vi "String.Merge data from 2 lists.vi"(8 "New Values":string[](array[string]), 9 "New Names":string[](array[string]), 11 "Names":string[](array[string])) -> (1 "Added Names":bool, 2 "Values Out":string[](array[string]), 3 "Names Out":string[](array[string]))   [LabVIEW 2019]
panel:
  out "appended array":string[](array[string])
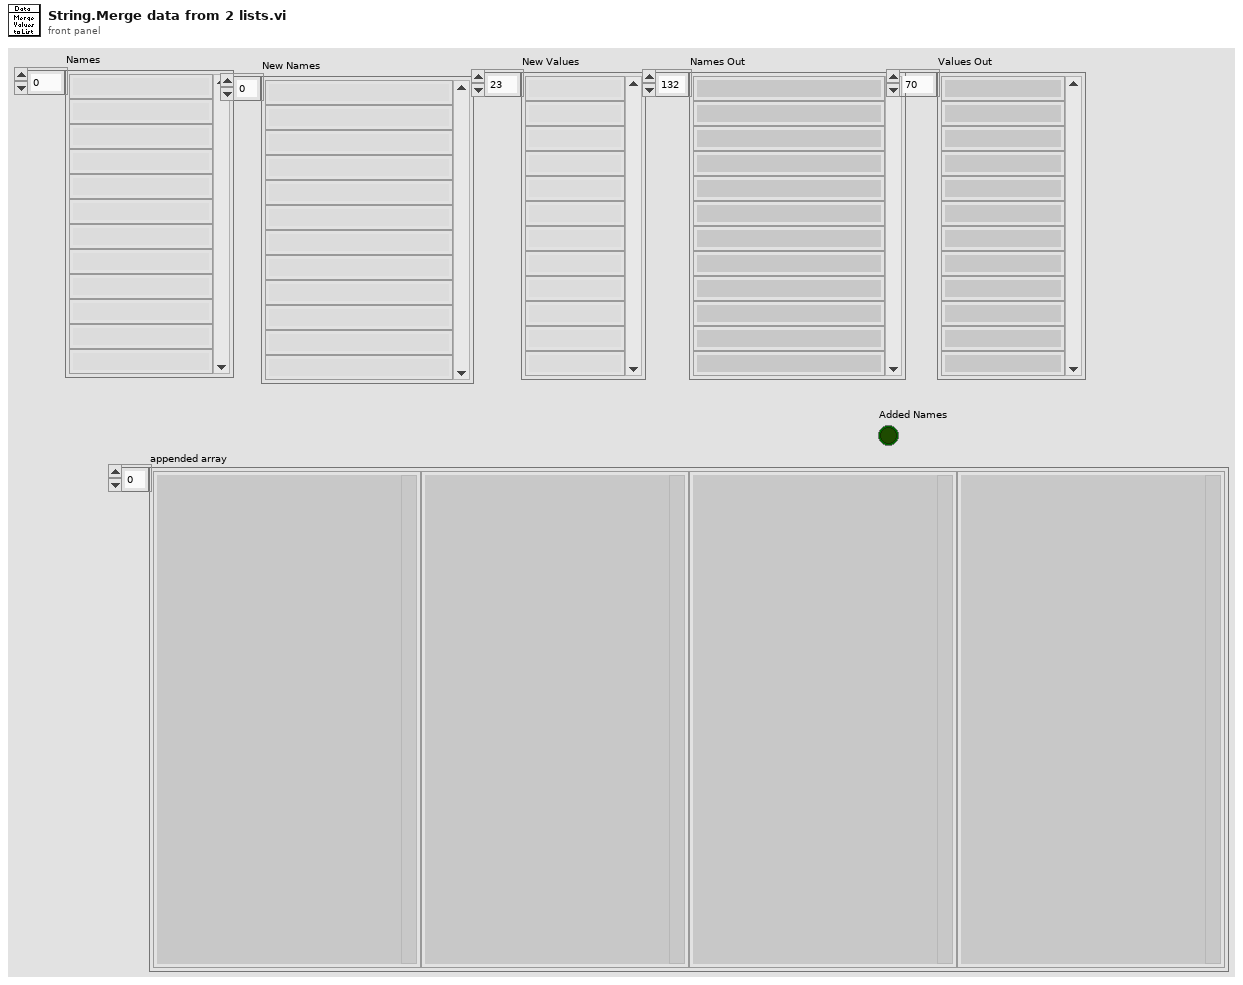
[diagram p1: front panel]
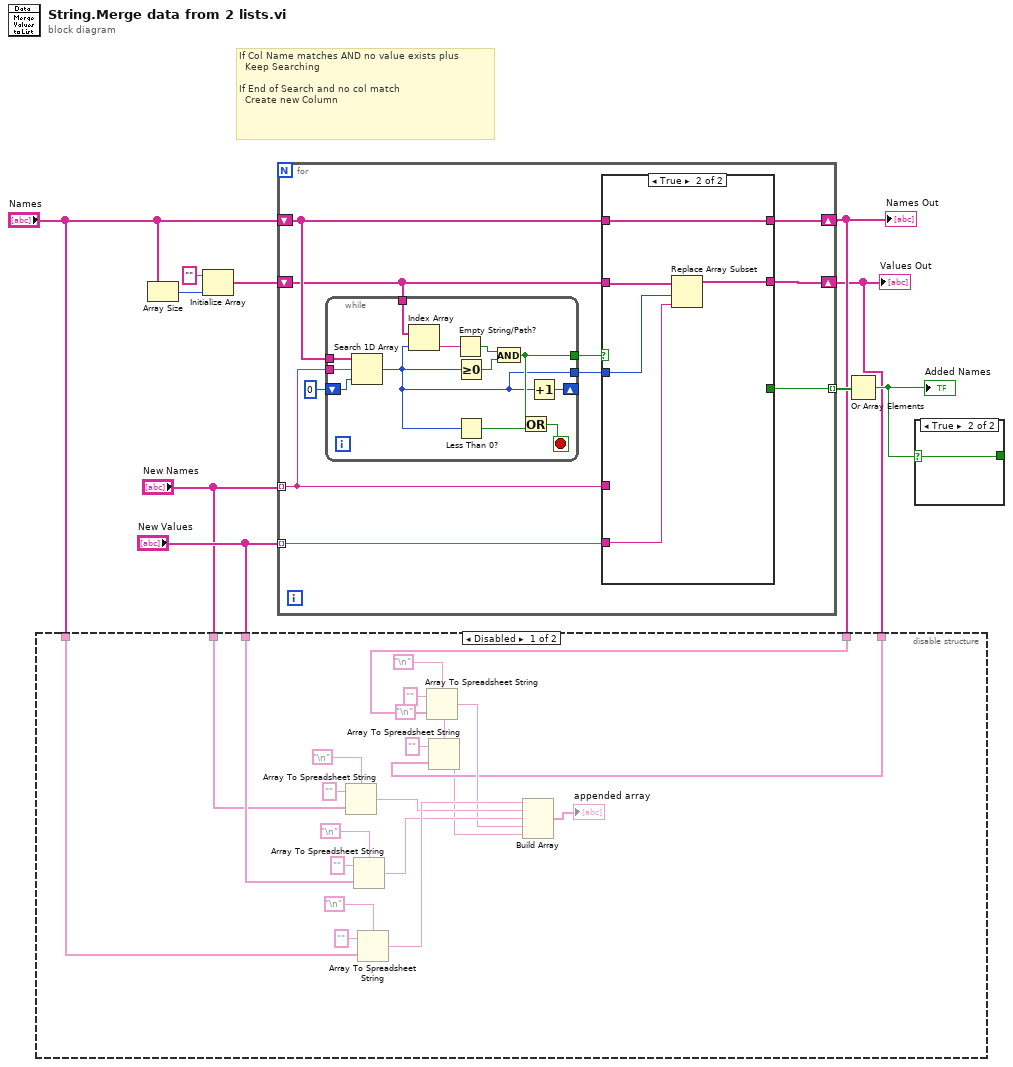
[diagram p0: block diagram]
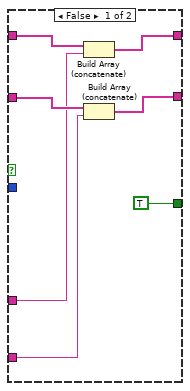
[diagram p4: hidden frame]
diagram:
  # "If Col Name matches AND no value exists plus\n  Keep Searching\n\nIf End of Search and no col match   \n  Create new Column"
  n1 = Array Size(array="Names") -> (size(s)=w10:i32)
  n2 = Initialize Array("", w10) -> (w8:string[])
  n3 = for {
    tunnel: "New Names" -> [w20] mode=indexing
    shift-right: [w18] -> w2
    shift-left: "Names" -> [w19]
    tunnel: "New Values" -> [w17] mode=indexing
    shift-right: [w16] -> w1
    shift-left: w8 -> [w15]
    tunnel: [w11] -> w7 mode=indexing
    n4 = while {
      tunnel: w20 -> [w32]
      tunnel: w19 -> [w31]
      tunnel: w15 -> [w30]
      tunnel: [w24] -> w14
      shift-right: [w22] -> _
      shift-left: 0 ("index of element") -> [w23]
      tunnel: [w21] -> w12
      stop <- w26 stop-if-true
      n5 = Search 1D Array(1D array=w31, element=w32, start index (0)=w23) -> (index of element=w21:i32)
      n6 = Index Array(array=w30, index=w21) -> (element=w29:string)
      n7 = Empty String/Path?(string/path=w29) -> (empty?=w28:bool)
      n8 = Greater Or Equal To 0?(x=w21) -> (x >= 0?=w27:bool)
      n9 = Less Than 0?(x=w21) -> (x < 0?=w25:bool)
      n10 = And(x=w28, y=w27) -> (x .and. y?=w24:bool)
      n11 = Or(x=w24, y=w25) -> (x .or. y?=w26:bool)
      n12 = Increment(x=w21) -> (x+1=w22:i32)
    }
    n13 = case shown="True" w14 {
      tunnel: w20 -> [w36 _]
      tunnel: w19 -> [w39 w43]
      tunnel: [w38 w43] -> w18
      tunnel: w15 -> [w37 w44]
      tunnel: w17 -> [w35 w41]
      tunnel: [w34 w42] -> w16
      tunnel: w12 -> [_ w40]
      tunnel: [TRUE _] -> w11
      frame False {
        n14 = Build Array (concatenate)(w39, w36) -> (w38:string[])
        n15 = Build Array (concatenate)(w37, w35) -> (w34:string[])
      }
      frame True {
        n16 = Replace Array Subset(array=w44, new element=w41, index=w40) -> (w42:string[])
      }
    }
  }
  "Names Out" <- w2
  "Values Out" <- w1
  n17 = disable-structure shown="Disabled" {
    disable-tunnel: "New Values" -> [w65 _]
    disable-tunnel: "New Names" -> [w60 _]
    disable-tunnel: "Names" -> [w57 _]
    disable-tunnel: w2 -> [w49 _]
    disable-tunnel: w1 -> [w46 _]
    frame Disabled {
      n18 = Array To Spreadsheet String(delimiter (Tab)="\n", array=w60, 3:"" ("format string")) -> (spreadsheet string=w53:string)
      n19 = Array To Spreadsheet String(delimiter (Tab)="\n", array=w65, 3:"" ("format string")) -> (spreadsheet string=w54:string)
      n20 = Array To Spreadsheet String(delimiter (Tab)="\n", array=w57, 3:"" ("format string")) -> (spreadsheet string=w55:string)
      n21 = Array To Spreadsheet String(delimiter (Tab)="\n", array=w49, 3:"" ("format string")) -> (spreadsheet string=w50:string)
      n22 = Array To Spreadsheet String(delimiter (Tab)="\n", array=w46, 3:"" ("format string")) -> (spreadsheet string=w45:string)
      n23 = Build Array(w55, w53, w54, w50, w45) -> (→"appended array":string[])
    }
    frame Enabled {
    }
  }
  n24 = Or Array Elements(Boolean array=w7) -> (logical OR=w6:bool)
  "Added Names" <- w6
  n25 = case shown="True" w6 {
    selector: w6 -> [_ w66]
    tunnel: [_ w66] -> _
    frame False {
    }
    frame True {
    }
  }
